vi "ExCenterStripADC.vi"() -> ()   [LabVIEW 2010]
panel:
  in  "Readout Port":i32=-1 min=-1 step=1
  in  "ADC Offset":i32=-1 min=-1 step=1
  in  "ADC Gain":i32=-1 min=-1 step=1
  in  "ADC speed":i32=-2 min=-3 step=1
  out "Strip":sgl[](graph)
  in  "Temperature":dbl=-10.0 format="%.2f"
  in  "Exposure":dbl min=0.0 step=0.001 format="%.3f"
  in  "stop":bool
  out "error out":errorcluster
  in  "error in (no error)":errorcluster
  # "ExCenterStrip:\nThis example selects the center strip of the CCD for the ROI and then \ncollects the data using circular buffers. It collects data until the stop \nbutton is pushed."
  # "For Slowest ADC speed set this to -3\nFor Fastest ADC speed set this to -2\nTo use current ADC speed don't  hook up or use -1\notherwise put speed in as kHz"
  # "To use current gain don't hook up or set to -1"
  # "To use current gain don't hook up or set to -1"
  # "To use current gain don't hook up or set to -1"
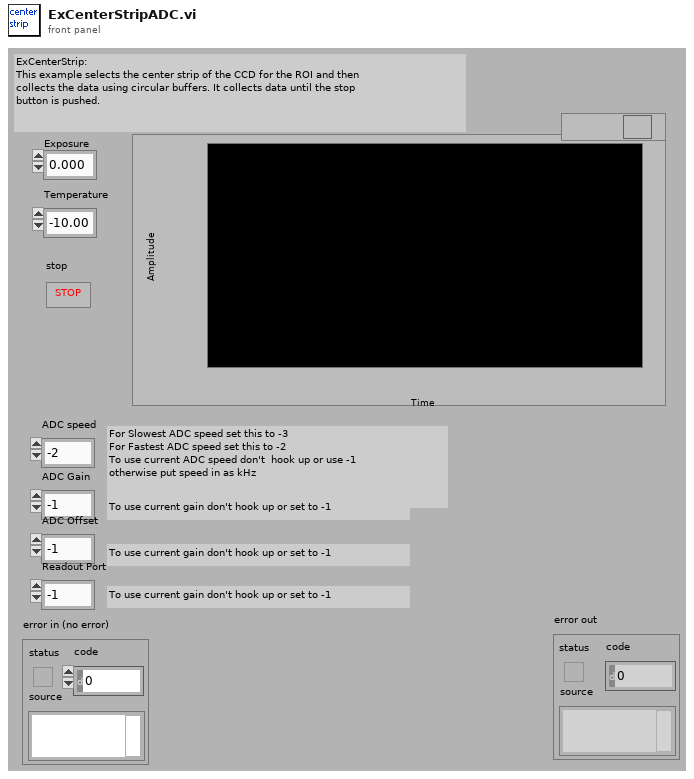
[diagram p1: front panel]
types:
  T1 = cluster{"Acquire / focus mode \n1 is Sync circualar buffers":i32, "Exposure":dbl, "Number of Images":i32, "Number of software\naccumulations":i32}
  T2 = cluster{"Camera Handle":u32, "Pulser Handle":u32, "File Handle":u32, "Display Handle":u32, "Image Handle":u32}
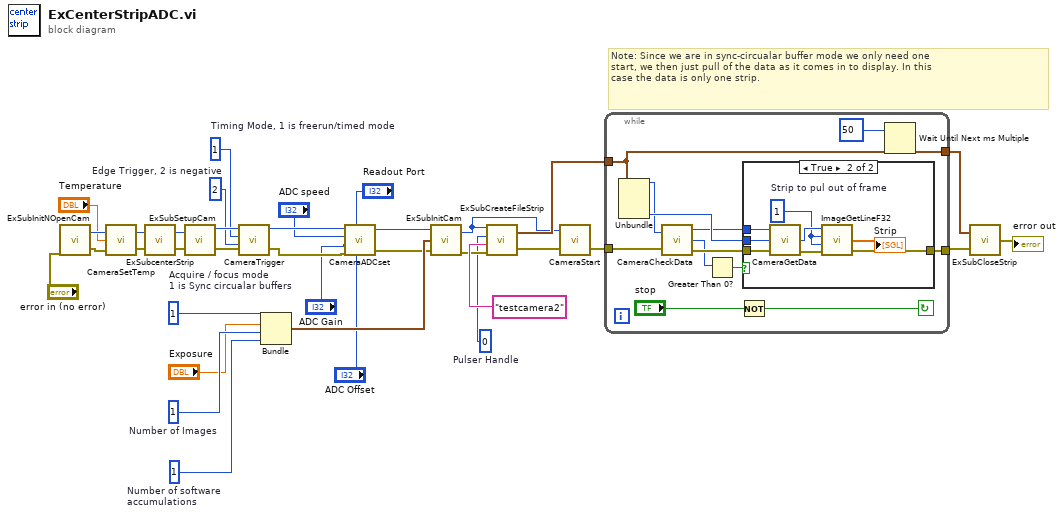
[diagram p0: block diagram]
diagram:
  w19 = 2  # Edge Trigger, 2 is negative
  w20 = 1  # Timing Mode, 1 is freerun/timed mode
  w27 = 0  # Pulser Handle
  w33 = 1  # Number of Images
  w34 = 1  # Acquire / focus mode  1 is Sync circualar buffers
  w32 = 1  # Number of software accumulations
  # "Note: Since we are in sync-circualar buffer mode we only need one\nstart, we then just pull of the data as it comes in to display. In this \ncase the data is only one strip."
  n1 = call "ExSubInitNOpenCam.vi"("error in (no error)"="error in (no error)") -> ("Camera Handle"=w11:u32, "error out"=w10:errorcluster)
  n2 = call <userlib>:"CameraSetTemp.vi"("error in (no error)"=w10, "Temperature"="Temperature", "Camera Handle"=w11) -> ("error out"=w12:errorcluster, "Camera Handle"=w13:u32)
  n3 = call "ExSubcenterStrip.vi"("error in (no error)"=w12, "Camera Handle"=w13) -> ("error out"=w15:errorcluster, "Camera Handle"=w14:u32)
  n4 = call "ExSubSetupCam.vi"("error in (no error)"=w15, "Camera Handle"=w14) -> ("error out"=w18:errorcluster, "Camera Handle"=w21:u32)
  n5 = call <userlib>:"CameraTrigger.vi"("error in"=w18, "Trigger Edge"=w19, "Timing Mode"=w20, "Camera Handle"=w21) -> ("error out"=w8:errorcluster, "Camera Handle"=w5:u32)
  n6 = Bundle("Acquire / focus mode \n1 is Sync circualar buffers"=w34, "Exposure"="Exposure", "Number of Images"=w33, "Number of software\naccumulations"=w32) -> (w29:T1)  [unwired: 1 in]
  n7 = call <userlib>:"CameraADCset.vi"("ADC offset"="ADC Offset", "Read Out port"="Readout Port", "error in (no error)"=w8, "ADC Gain"="ADC Gain", "ADC Speed"="ADC speed", "Camera Handle"=w5) -> ("error out"=w7:errorcluster, "Camera Handle"=w6:u32)
  n8 = call "ExSubInitCam.vi"("error in (no error)"=w7, "Camera Information"=w29, "Camera Handle"=w6) -> ("error out"=w28:errorcluster, "Camera Handle"=w25:u32)
  n9 = call "ExSubCreateFileStrip.vi"("error in (no error)"=w28, "File and Display Name"="testcamera2", "Pulser Handle"=w27, "Camera Handle"=w25) -> ("error out"=w16:errorcluster, "Handles Out"=w26:T2)
  n10 = call <userlib>:"CameraStart.vi"("error in"=w16, "Camera Handle"=w25) -> ("error out"=w17:errorcluster)  [unwired: 1 out]
  n11 = while {
    tunnel: w26 -> [w44]
    tunnel: w17 -> [w43]
    tunnel: [w41] -> w23
    tunnel: [w44] -> w24
    stop <- w45 continue-if-true
    n12 = Unbundle(w44) -> ("Camera Handle"=w39:u32, "Image Handle"=w40:u32)  [unwired: 3 out]
    n13 = call <userlib>:"CameraCheckData.vi"("Camera Handle"=w39, "error in"=w43) -> ("Camera Handle"=w38:u32, "Number Of Frames Available"=w36:i32, "error out"=w42:errorcluster)
    n14 = Greater Than 0?(x=w36) -> (x > 0?=w37:bool)
    n15 = Not(x="stop") -> (.not. x?=w45:bool)
    n16 = case shown="True" w37 {
      tunnel: w42 -> [w48 w55]
      tunnel: [w48 w53] -> w41
      tunnel: w40 -> [_ w50]
      tunnel: w38 -> [_ w49]
      frame False {
      }
      frame True {
        w51 = 1  # Strip to pul out of frame
        n17 = call <userlib>:"CameraGetData.vi"("error in"=w55, "Data Handle"=w50, "Camera Handle"=w49) -> ("error out"=w54:errorcluster, "Data Handle"=w52:u32)  [unwired: 1 out]
        n18 = call <userlib>:"ImageGetLineF32.vi"("error in"=w54, "Z Position"=w51, "Y Position"=w51, "Data Handle"=w52) -> ("error out"=w53:errorcluster, "Array F32"=→"Strip":sgl[])  [unwired: 1 out]
      }
    }
    n19 = Wait Until Next ms Multiple(millisecond multiple=50) -> ()  [unwired: 1 out]
  }
  n20 = call "ExSubCloseStrip.vi"("error in (no error)"=w23, "Handles In"=w24) -> ("error out"=→"error out":errorcluster)
